vi "Tester Sequence.vi"() -> ()   [LabVIEW 2014, in "CAP-USB-1.lvlib"]
uses:
  CAP-USB-1.lvlib
  CAP-USB-1Class/CAP-USB-1.lvclass
panel:
  out "Array":sgl[](array[numeric])
  out "error out 2":errorcluster
  in  "stop 2":bool
  out "Muestras por segundo":dbl
  out "Segundos":dbl
  out "TDX":sgl[][](array[numeric])
  out "Muestras":i32
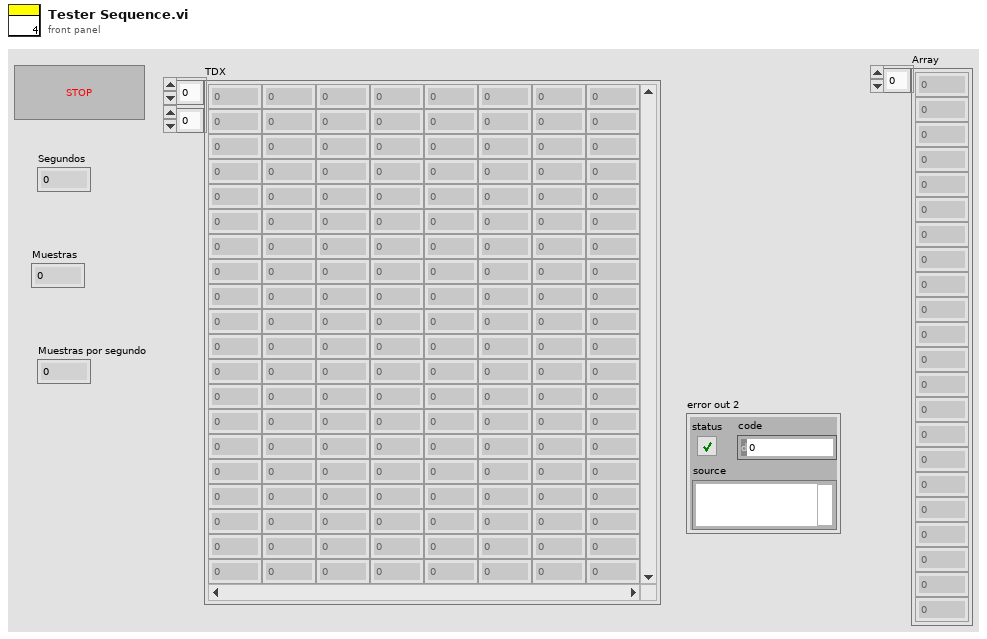
[diagram p1: front panel]
types:
  T1 = typedef "DriverMasterSync.lvlibp/WINFAS 2 Data Queue.lvlib/Control Data Cluster.ctl" = cluster{"Encoder":sgl, "DI":bool[], "DO":bool[]}
  T2 = typedef "DriverMasterSync.lvlibp/WINFAS 2 Data Queue.lvlib/Acquisition Data Cluster.ctl" = T3[]
  T3 = typedef "DriverMasterSync.lvlibp/WINFAS 2 Data Queue.lvlib/Acquisition Data 1 Sample Cluster.ctl" = cluster{"TDX":sgl[], "Encoder":sgl}
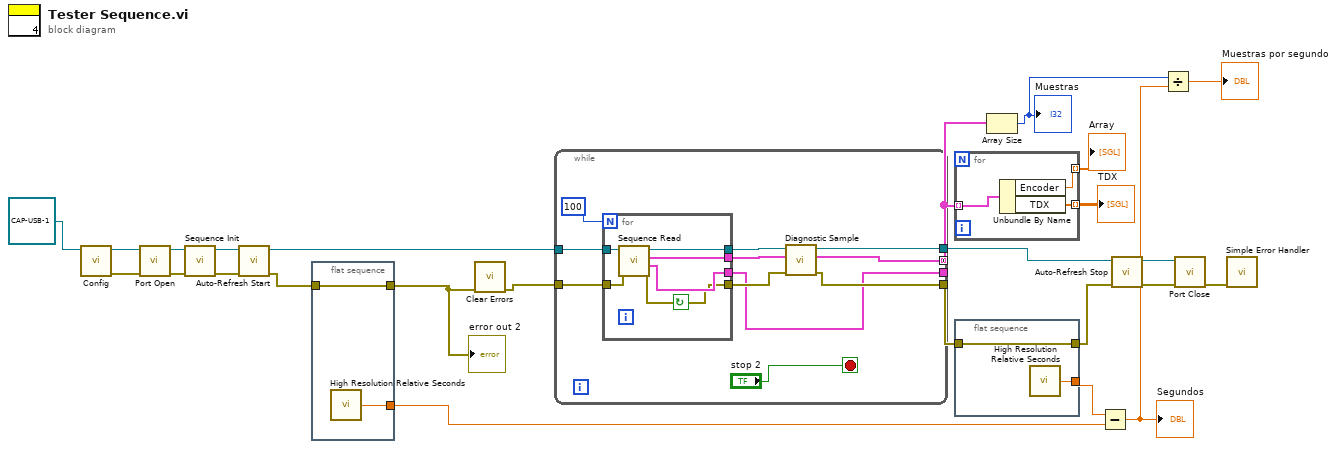
[diagram p0: block diagram]
diagram:
  n1 = call-dynamic "Config.vi"("CAP-USB-1 in"=refnum<class "CAP-USB-1.lvclass"> refnum) -> ("error out"=w24:errorcluster, "CAP-USB-1 out"=w11:refnum<class "CAP-USB-1.lvclass">)  [unwired: 8 in, 1 out]
  n2 = call-dynamic "Port Open.vi"("error in (no error)"=w24, "CAP-USB-1 in"=w11) -> ("error out"=w9:errorcluster, "CAP-USB-1 out"=w10:refnum<class "CAP-USB-1.lvclass">)  [unwired: 8 in]
  n3 = call-dynamic "Sequence Init.vi"("error in (no error)"=w9, "CAP-USB-1 in"=w10) -> ("error out"=w7:errorcluster, "CAP-USB-1 out"=w8:refnum<class "CAP-USB-1.lvclass">)  [unwired: 8 in]
  n4 = call-dynamic "Auto-Refresh Start.vi"("error in (no error)"=w7, "CAP-USB-1 in"=w8) -> ("error out"=w2:errorcluster, "CAP-USB-1 out"=w3:refnum<class "CAP-USB-1.lvclass">)  [unwired: 8 in]
  n5 = flat-sequence {
    tunnel: w2 -> [w27]
    tunnel: [w27] -> w5
    tunnel: [w26] -> w14
    frame #0 {
      n6 = call <vilib>:"High Resolution Relative Seconds.vi"() -> ("relative seconds"=w26:dbl)
    }
  }
  n7 = call <vilib>:"Clear Errors.vi"("error in (no error)"=w5) -> ("error out"=w4:errorcluster)  [unwired: 5 in, 1 out]
  n8 = while {
    tunnel: [w29] -> w6
    tunnel: [w33] -> w17
    tunnel: [w31] -> w13 mode=concatenating
    tunnel: [w28] -> _
    tunnel: w4 -> [w38]
    tunnel: w3 -> [w37]
    stop <- "stop 2" stop-if-true
    n9 = for {
      N: 100 -> [_]
      tunnel: [w42] -> w28
      tunnel: [w40] -> w32
      tunnel: w38 -> [w44]
      tunnel: [w39] -> w30
      tunnel: w37 -> [w43]
      tunnel: [w41] -> w34
      stop <- w39 continue-if-true
      n10 = call-dynamic "Sequence Read.vi"("error in (no error)"=w44, "CAP-USB-1 in"=w43) -> ("error out"=w39:errorcluster, "Control Data"=w42:T1, "Acquisition Data"=w40:T2, "CAP-USB-1 out"=w41:refnum<class "CAP-USB-1.lvclass">)  [unwired: 6 in]
    }
    n11 = call-dynamic "Diagnostic Sample.vi"("error in (no error)"=w30, "Acquisition Data"=w32, "CAP-USB-1 in"=w34) -> ("error out"=w29:errorcluster, "Acquisition Data"=w31:T2, "CAP-USB-1 out"=w33:refnum<class "CAP-USB-1.lvclass">)  [unwired: 6 in]
  }
  n12 = for {
    tunnel: w13 -> [w47] mode=indexing
    tunnel: [w46] -> w16 mode=indexing
    tunnel: [w45] -> w1 mode=indexing
    n13 = Unbundle By Name(w47) -> ("Encoder"=w45:sgl, "TDX"=w46:sgl[])
  }
  "TDX" <- w16
  "Array" <- w1
  n14 = flat-sequence {
    tunnel: w6 -> [w49]
    tunnel: [w49] -> w12
    tunnel: [w48] -> w15
    frame #0 {
      n15 = call <vilib>:"High Resolution Relative Seconds.vi"() -> ("relative seconds"=w48:dbl)
    }
  }
  n16 = Array Size(array=w13) -> (size(s)=w19:i32)
  "Muestras" <- w19
  n17 = Subtract(x=w15, y=w14) -> (x-y=w21:dbl)
  "Segundos" <- w21
  n18 = call-dynamic "Auto-Refresh Stop.vi"("error in (no error)"=w12, "CAP-USB-1 in"=w17) -> ("error out"=w23:errorcluster, "CAP-USB-1 out"=w25:refnum<class "CAP-USB-1.lvclass">)  [unwired: 8 in]
  n19 = Divide(x=w19, y=w21) -> (x/y=→"Muestras por segundo":dbl)
  n20 = call-dynamic "Port Close.vi"("error in (no error)"=w23, "CAP-USB-1 in"=w25) -> ("error out"=w18:errorcluster)  [unwired: 8 in, 1 out]
  n21 = call <vilib>:"Simple Error Handler.vi"("error in (no error)"=w18) -> ()  [unwired: 4 in, 5 out]
  "error out 2" <- w5
